vi "Format T-SQL Datetime2 To Timestamp.vi"(11 "datetime2":string) -> (3 "Time":timestamp)   [LabVIEW 2015, in "Utility.lvlib"]
uses:
  Utility.lvlib
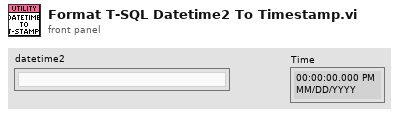
[diagram p1: front panel]
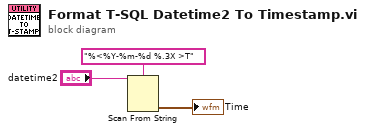
[diagram p0: block diagram]
diagram:
  n1 = Scan From String(format string="%<%Y-%m-%d %.3X >T", input string="datetime2") -> (output 1=→"Time":timestamp)  [unwired: 3 in, 3 out]
